vi "Test program 3.vi"() -> ()   [LabVIEW 2013, in "Keithly user program.lvlib"]
uses:
  Keithly user program.lvlib
panel:
  in  "stop":bool
  out "Waveform Chart":dbl[](graph)
  out "2182 -A Params":T1={"Auto Range?"=FALSE, "Man / Selected\n        Range"=0, "Enable Digital\n       Filter?"=FALSE, "Filter Type"=0, "Filter Count"=1, "      Filter\nWindow (%)"=0.01, "Enable Analog\n       Filter?"=FALSE, "NPLCs"=5} {"NPLCs" min=1 max=10; "Filter\nWindow (%)" min=0.01 max=10.0 step=0.01 format="%.2f"; "Filter Count" min=1 max=100; "Filter Type" items=["Movin", "Repeat"]; "Man / Selected\n        Range" items=["10mV", "100mV", "1V", "10V", "100V"]}
  in  "2182 -A Params In":T2={"Auto Range?"=FALSE, "Man / Selected\n       Range"=enum."10mV", "Enable Digital\n       Filter?"=FALSE, "Filter Type"=enum."Movin", "Filter Count"=1, "      Filter\nWindow (%)"=0.01, "Enable Analog\n       Filter?"=FALSE, "NPLCs"=5} {"NPLCs" min=1 max=10; "Filter\nWindow (%)" min=0.01 max=10.0 step=0.01 format="%.2f"; "Filter Count" min=1 max=100}
  in  "622x Resource In":refnum<visa-resource-name>
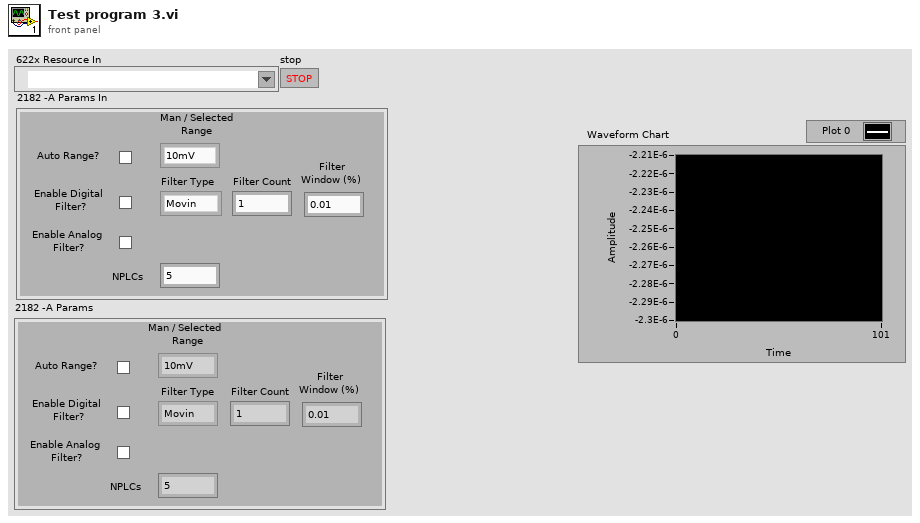
[diagram p1: front panel]
types:
  T1 = cluster{"Auto Range?":bool, "Man / Selected\n        Range":u16, "Enable Digital\n       Filter?":bool, "Filter Type":u16, "Filter Count":u32, "      Filter\nWindow (%)":dbl, "Enable Analog\n       Filter?":bool, "NPLCs":u32}
  T2 = cluster{"Auto Range?":bool, "Man / Selected\n       Range":enum16{"10mV", "100mV", "1V", "10V", "100V"}, "Enable Digital\n       Filter?":bool, "Filter Type":enum16{"Movin", "Repeat"}, "Filter Count":u32, "      Filter\nWindow (%)":dbl, "Enable Analog\n       Filter?":bool, "NPLCs":u32}
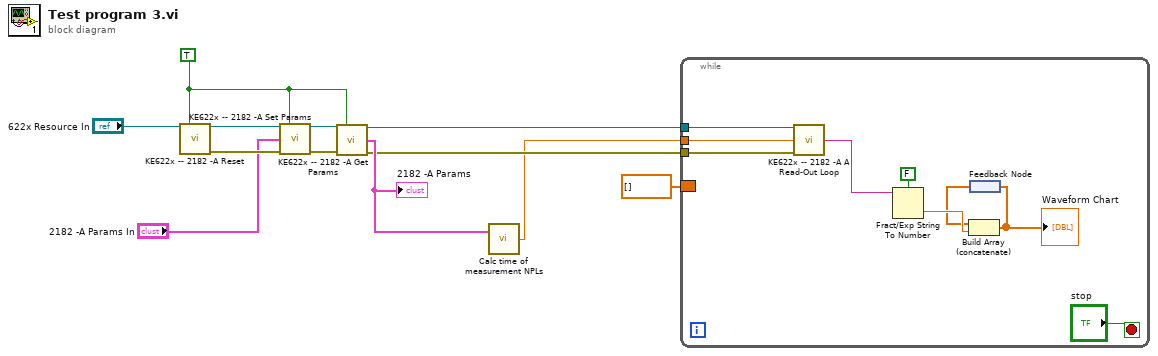
[diagram p0: block diagram]
diagram:
  w7 = TRUE ("Check For SCPI Errors? (T)")
  n1 = call "KE622x -- 2182 -A Reset.vi"("622x Resource In"="622x Resource In", "Check For SCPI Errors? (T)"=w7) -> ("622x Resource Out (dupl)"=w11:refnum<visa-resource-name>, "error out"=w10:errorcluster)  [unwired: 12 in]
  n2 = call "KE622x -- 2182 -A Set Params.vi"("622x Resource In"=w11, "Check For SCPI Errors? (T)"=w7, "2182 -A Params In"="2182 -A Params In", "error in (no error)"=w10) -> ("622x Resource Out (dupl)"=w9:refnum<visa-resource-name>, "error out"=w8:errorcluster)  [unwired: 10 in]
  n3 = call "KE622x -- 2182 -A Get Params.vi"("622x Resource In"=w9, "Check For SCPI Errors? (T)"=w7, "error in (no error)"=w8) -> ("622x Resource Out (dupl)"=w4:refnum<visa-resource-name>, "2182 -A Params"=w5:T1, "error out"=w3:errorcluster)  [unwired: 10 in]
  "2182 -A Params" <- w5
  n4 = call "Calc time of measurement NPLs.vi"("2182 -A Params"=w5) -> ("Time of one measurement"=w2:dbl)  [unwired: 1 in]
  n5 = while {
    tunnel: w4 -> [w21]
    tunnel: w3 -> [w20]
    tunnel: w2 -> [w19]
    border: dbl[] [] -> [_]
    stop <- "stop" stop-if-true
    n6 = call "KE622x -- 2182 -A A Read-Out Loop.vi"("622x Resource In"=w21, "Time of one measurement"=w19, "error in (no error)"=w20) -> ("2182-A Reponse String"=w18:string)  [unwired: 10 in, 2 out]
    n7 = Fract/Exp String To Number(use system decimal point (T)=FALSE, string=w18) -> (number=w16:dbl)  [unwired: 2 in, 1 out]
    n8 = feedback #1() -> (w15:dbl[])
    n9 = Build Array (concatenate)(w15, w16) -> (w14:dbl[])
    "Waveform Chart" <- w14
    n10 = feedback-in #1(w14) -> ()
  }
